vi "InitMODEL.vi"(8 "error in (no error)":errorcluster, 11 "CONTROLLER in":refnum<class "CONTROLLER.lvclass">) -> (0 "error out":errorcluster, 3 "CONTROLLER out":refnum<class "CONTROLLER.lvclass">)   [LabVIEW 2013, in "CONTROLLER.lvclass"]
uses:
  CONTROLLER.lvclass
  Model/base/MODEL.lvclass
  CONTROLLER.lvclass/CONTROLLER.ctl
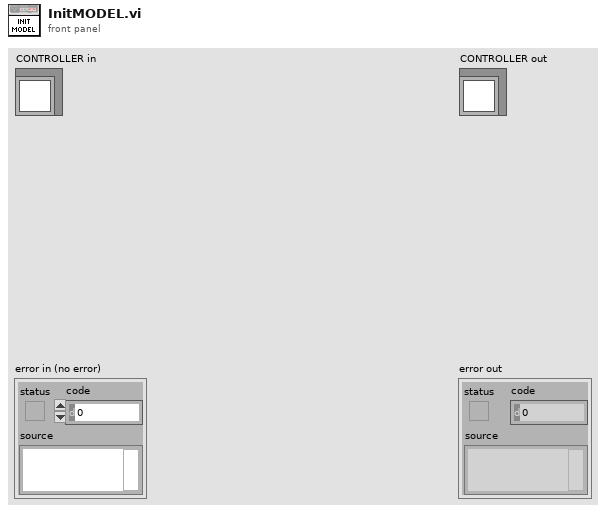
[diagram p1: front panel]
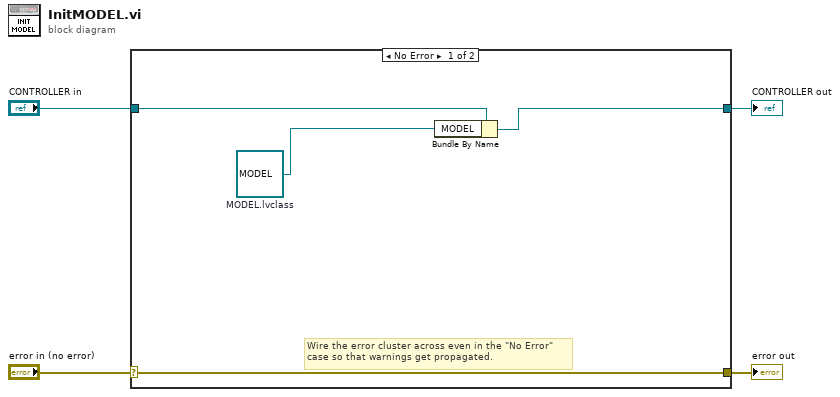
[diagram p0: block diagram]
diagram:
  n1 = case shown="No Error" "error in (no error)" {
    selector: "error in (no error)" -> [w8 w10]
    tunnel: [w8 w10] -> w3
    tunnel: [w6 w9] -> w1
    tunnel: "CONTROLLER in" -> [w7 w9]
    frame No Error {
      w5 = refnum<class "MODEL.lvclass"> refnum  # MODEL.lvclass
      # "Wire the error cluster across even in the \"No Error\"\ncase so that warnings get propagated."
      n2 = Bundle By Name(cluster=w7, "MODEL"=w5) -> (w6:refnum<class "CONTROLLER.lvclass">)
    }
    frame Error {
    }
  }
  "error out" <- w3
  "CONTROLLER out" <- w1
